vi "GetPressureData.vi"(9 "PressureSensorID":u8[](array[numeric]), 10 "inputCANData":T1[](array[typedef]) {"payload" format="%x"; "timestamp" format="%<%.7X\n%x>T"; "type" items=["CAN Data"=0, "CAN Remote"=1, "CAN Bus Error"=2, "CAN 2.0 Data"=8, "CAN FD Data"=16, "CAN FD+BRS Data"=24, "J1939 Data"=192, "Delay"=224, "Log Trigger"=225, "Start Trigger"=226]; "identifier" format="%x"}) -> (2 "outputPressureData":dbl[](array[numeric]))   [LabVIEW 2020]
uses:
  <vilib>/xnet/xnet.llb/XNET Frame CAN.ctl
  <vilib>/xnet/xnet.llb/XNET Frame Type CAN.ctl
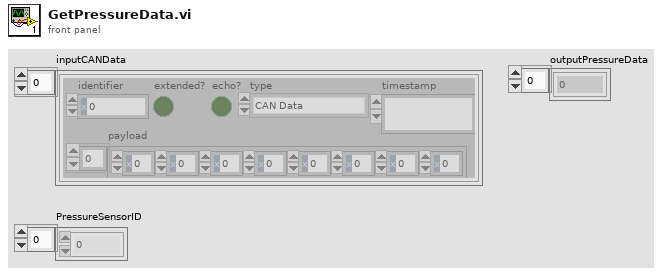
[diagram p1: front panel]
types:
  T1 = typedef "XNET Frame CAN.ctl" = cluster{"timestamp":timestamp, "payload":u8[], "identifier":u32, "type":T2, "extended?":bool, "echo?":bool}
  T2 = typedef "XNET Frame Type CAN.ctl" = u8
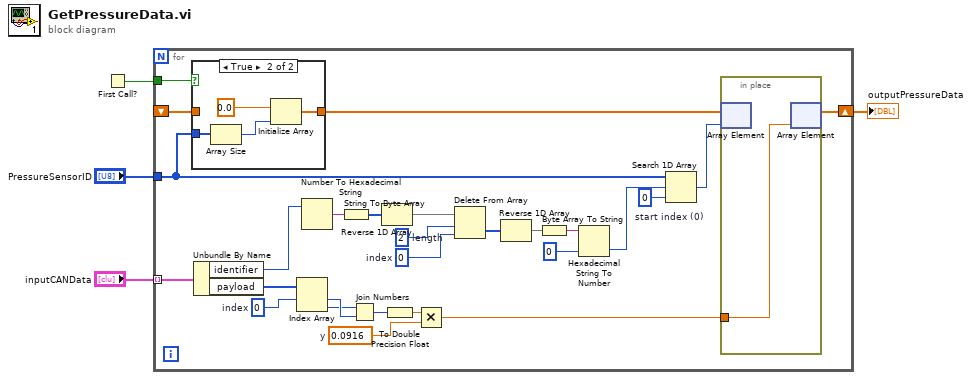
[diagram p0: block diagram]
diagram:
  n1 = First Call?() -> (First Call?: T/F=w1:bool)
  n2 = for {
    tunnel: "inputCANData" -> [w31] mode=indexing
    tunnel: "PressureSensorID" -> [w7]
    shift-right: [w10] -> w2
    shift-left: _ -> [w5]
    tunnel: w1 -> [w8]
    w9 = 0  # index
    w17 = 2  # length
    w16 = 0  # start index (0)
    w25 = 0.0916  # y
    w30 = 0  # index
    n3 = case shown="True" w8 {
      tunnel: w7 -> [_ w35]
      tunnel: [w32 w33] -> w6
      tunnel: w5 -> [w32 _]
      frame False {
      }
      frame True {
        n4 = Array Size(array=w35) -> (size(s)=w34:i32)
        n5 = Initialize Array "Initialize Array"(0.0 ("element"), w34) -> (w33:dbl[])
      }
    }
    n6 = Unbundle By Name(w31) -> ("identifier"=w15:u32, "payload"=w13:u8[])
    n7 = Index Array "Index Array"(array=w13, index #1=w30) -> (element #1=w29:u8, element #2=w28:u8)  [unwired: 1 in]
    n8 = Number To Hexadecimal String(2:w15) -> (0:w18:string)  [unwired: 1 in]
    n9 = String To Byte Array(string=w18) -> (unsigned byte array=w19:u8[])
    n10 = Join Numbers(hi=w28, lo=w29) -> ((hi.lo)=w27:u16)
    n11 = Reverse 1D Array(array=w19) -> (reversed array=w20:u8[])
    n12 = To Double Precision Float(number=w27) -> (double precision float=w26:dbl)
    n13 = Multiply(x=w26, y=w25) -> (x*y=w11:dbl)
    n14 = Delete From Array "Delete From Array"(array=w20, length=w17, index=w9) -> (deleted portion=w21:u8[])  [unwired: 1 out]
    n15 = Reverse 1D Array(array=w21) -> (reversed array=w22:u8[])
    n16 = Byte Array To String(unsigned byte array=w22) -> (string=w23:string)
    n17 = Hexadecimal String To Number(string=w23, default (0uL)=u8 0 ("default (0 U32)")) -> (number=w24:u8)  [unwired: 1 in, 1 out]
    n18 = Search 1D Array(1D array=w7, element=w24, start index (0)=w16) -> (index of element=w12:i32)
    n19 = in-place {
      in-place-border: w11 -> [w37]
      n20 = in-place-array #1(w6, w12) -> ()  [unwired: 1 out]
      n21 = in-place-array #1(w37) -> (w10:dbl[])  [unwired: 1 out]
    }
  }
  "outputPressureData" <- w2
